vi "Reporting_proc_RMS_inycom.vi"(1 "Max RMS Ruedas":dbl[][](array[numeric])) -> (0 "String":string)   [LabVIEW 2015]
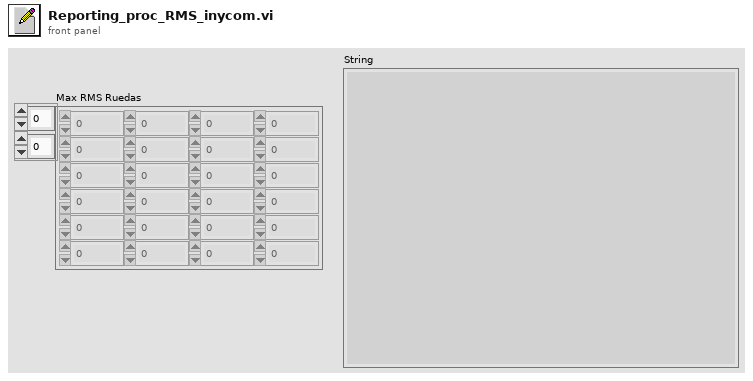
[diagram p1: front panel]
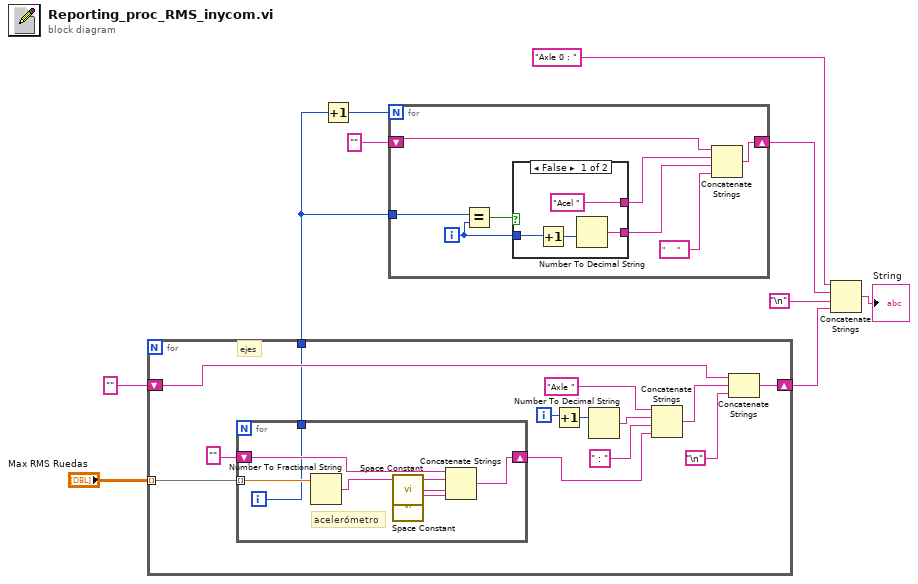
[diagram p0: block diagram]
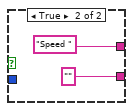
[diagram p2: hidden frame]
diagram:
  n1 = for {
    tunnel: "Max RMS Ruedas" -> [w23] mode=indexing
    shift-right: [w22] -> w4
    shift-left: "" -> [w21]
    tunnel: [w12] -> w1
    i -> [w18]
    # "ejes"
    n2 = for {
      tunnel: w23 -> [w30] mode=indexing
      shift-right: [w26] -> w14
      shift-left: "" -> [w25]
      tunnel: [w24] -> w12
      i -> [w24]
      # "acelerómetro"
      n3 = Number To Fractional String(number=w30) -> (F-format string=w29:string)  [unwired: 3 in]
      n4 = call <vilib>:"Space Constant.vi"() -> ("String"=w28:string)
      n5 = call <vilib>:"Space Constant.vi"() -> ("String"=w27:string)
      n6 = Concatenate Strings(w25, w29, w28, w27) -> (w26:string)
    }
    n7 = Increment(x=w18) -> (x+1=w17:i32)
    n8 = Number To Decimal String(number=w17) -> (decimal integer string=w16:string)  [unwired: 1 in]
    n9 = Concatenate Strings("Axle " ("string"), w16, " : " ("string"), w14) -> (w13:string)
    n10 = Concatenate Strings(w21, w13, "\n") -> (w22:string)
  }
  n11 = Increment(x=w1) -> (x+1=w2:i32)
  n12 = for {
    N: w2 -> [_]
    shift-right: [w36] -> w6
    shift-left: "" -> [w35]
    tunnel: w1 -> [w33]
    i -> [w34]
    n13 = Equal?(x=w33, y=w34) -> (x = y?=w32:bool)
    n14 = case shown="False" w32 {
      tunnel: ["Acel " ("string") "Speed " ("string")] -> w31
      tunnel: [w40 "" ("string")] -> w38
      tunnel: w34 -> [w39 _]
      frame False {
        n15 = Increment(x=w39) -> (x+1=w42:i32)
        n16 = Number To Decimal String(number=w42) -> (decimal integer string=w40:string)  [unwired: 1 in]
      }
      frame True {
      }
    }
    n17 = Concatenate Strings(w35, w31, w38, "      " ("string")) -> (w36:string)
  }
  n18 = Concatenate Strings("Axle 0 : " ("string"), w6, "\n", w4) -> (→"String":string)
